vi "7-19-19 Decreasing temp.vi"() -> ()   [LabVIEW 2016]
uses:
  <userlib>/Levylab/LV to ITX/LVtoITX.lvclass
  <vilib>/Analysis/NI_AALPro.lvlib
panel:
  out "G Vs Time 2":cluster{"Data":dbl[], "Data":dbl[]}(graph)
  in  "Path 2":path=path "G:/My Drive/Data/300 275 dec/SA40060.20190715.000007.dat"
  out "Data 2":dbl[][](array[numeric])
  out "dG/dt Vs Temp Normalized vs prev":cluster{"Data":dbl[], "Data":dbl[]}[](graph)
  out "dG/dt Vs Temp Normalized vs 275K":cluster{"Data":dbl[], "Data":dbl[]}[](graph)
  out "G Vs Time Fit":cluster{"Data":dbl[], "Data":dbl[]}[](graph)
  out "G Vs Time Cut":cluster{"Data":dbl[], "Data":dbl[]}[](graph)
  out "G Vs Temp":cluster{"Data":dbl[], "Data":dbl[]}[](graph)
  out "Data":dbl[][](array[numeric])
  out "G Vs Time":cluster{"Data":dbl[], "Data":dbl[]}[](graph)
  out "Wavenames":string[](array[string])
  in  "Path":path=path "G:/My Drive/Data/300 275 dec/SA40060.20190715.000007.dat"
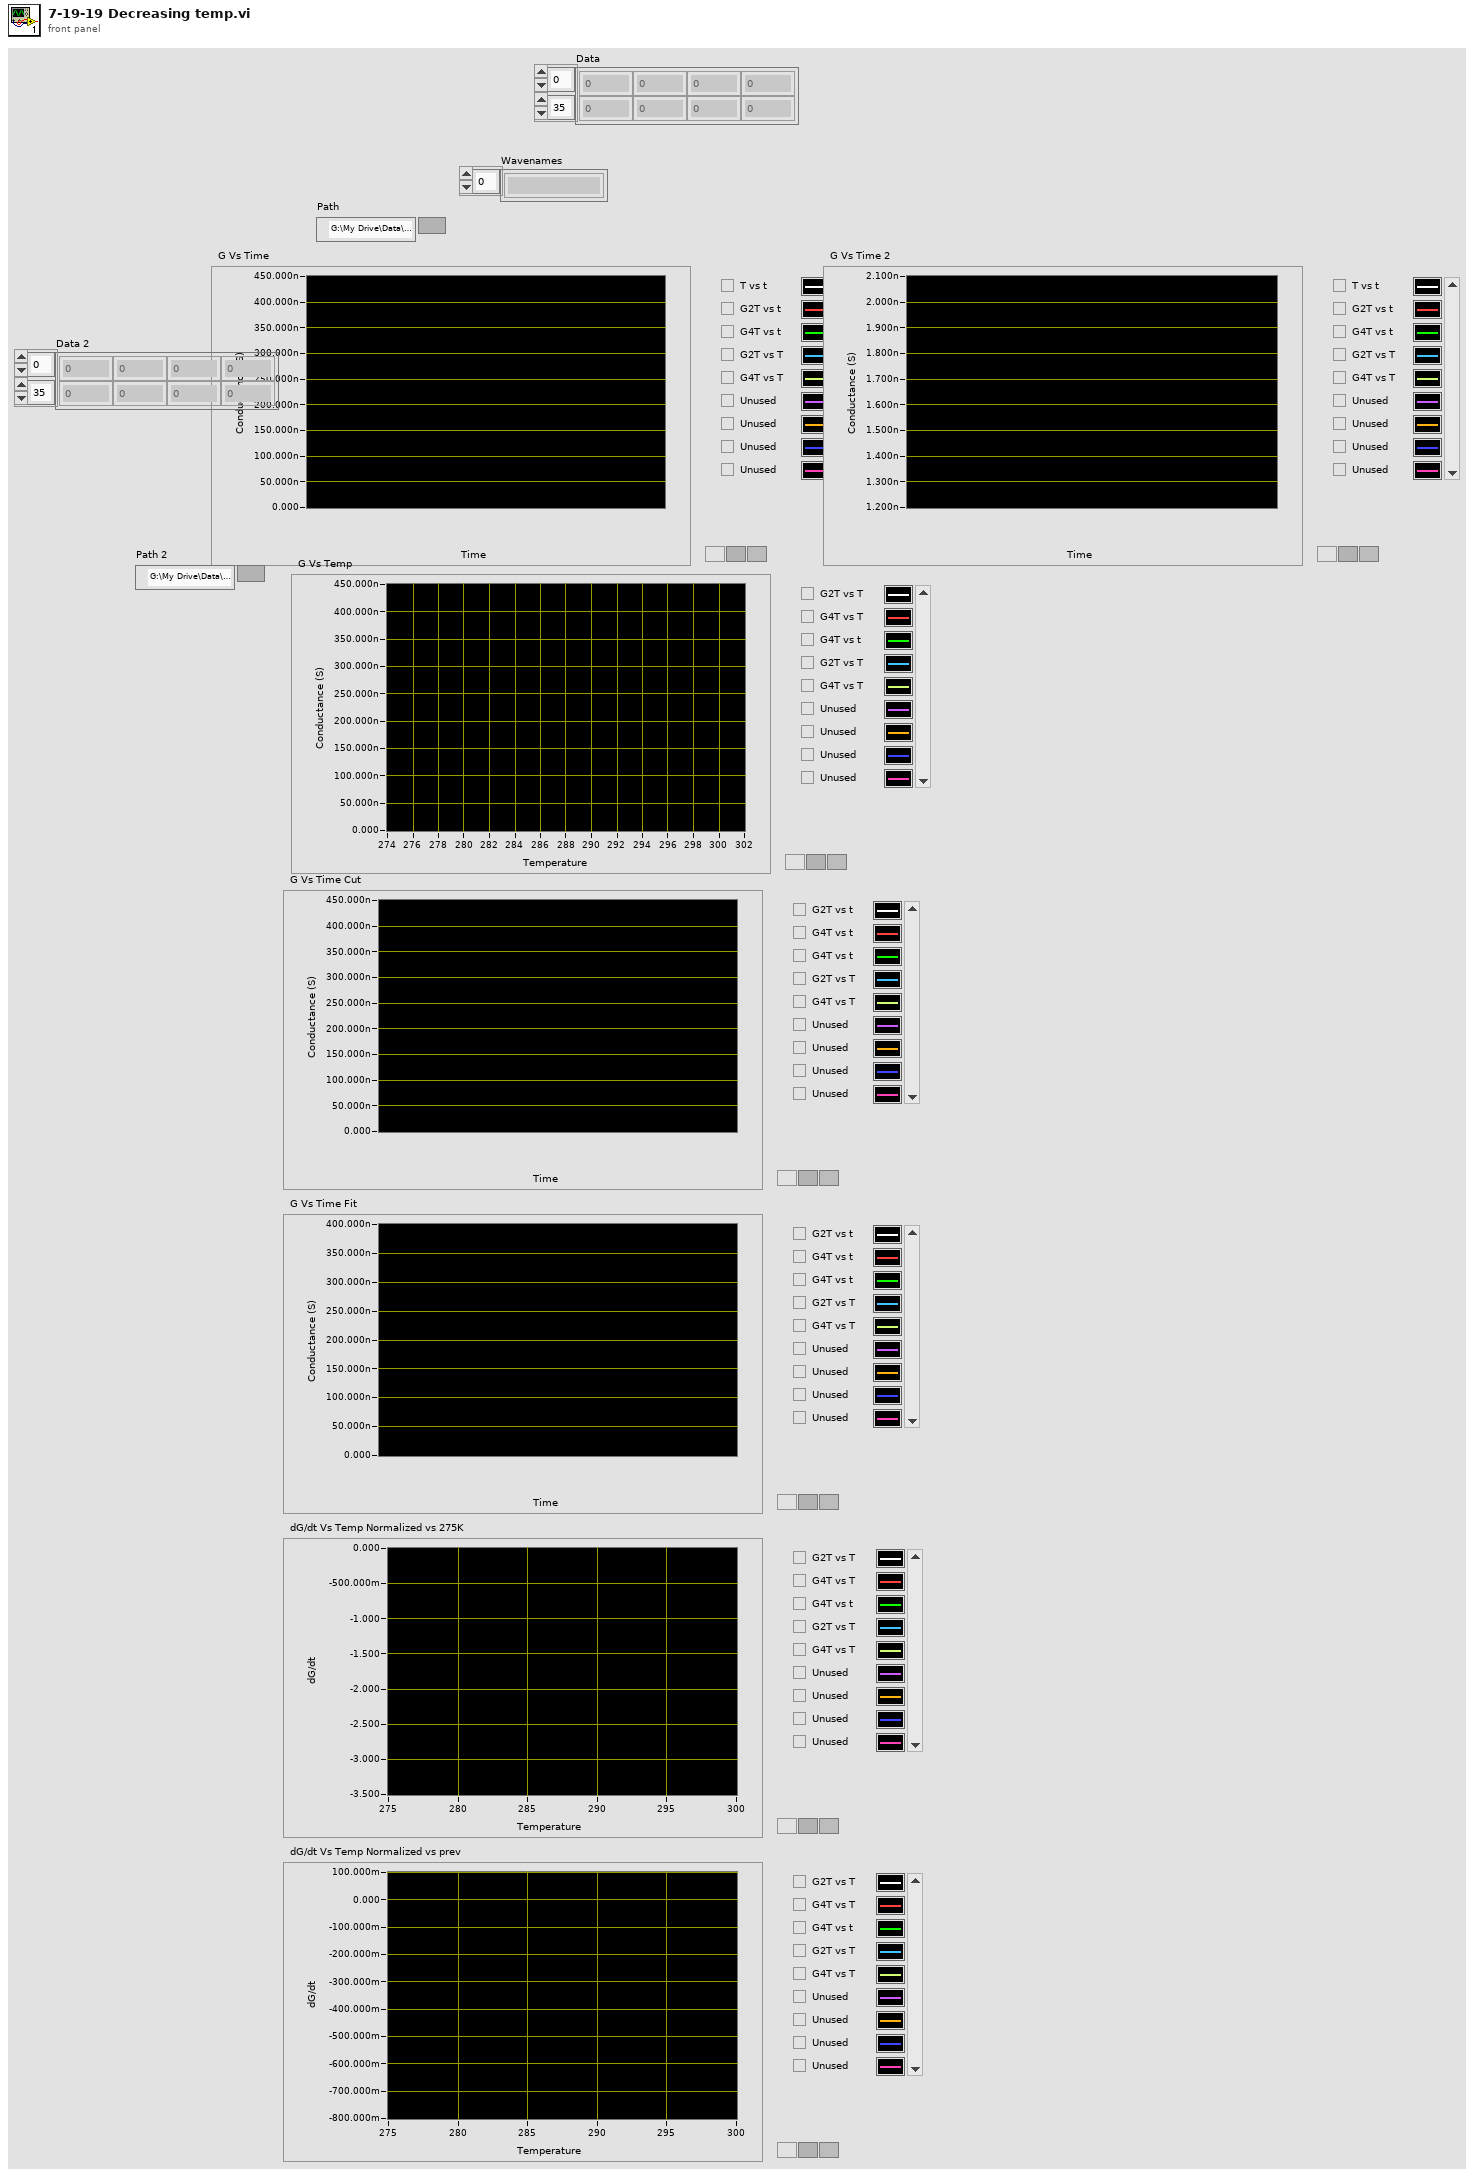
[diagram p1: front panel]
types:
  T1 = cluster{"slope min":dbl, "slope max":dbl, "intercept min":dbl, "intercept max":dbl}
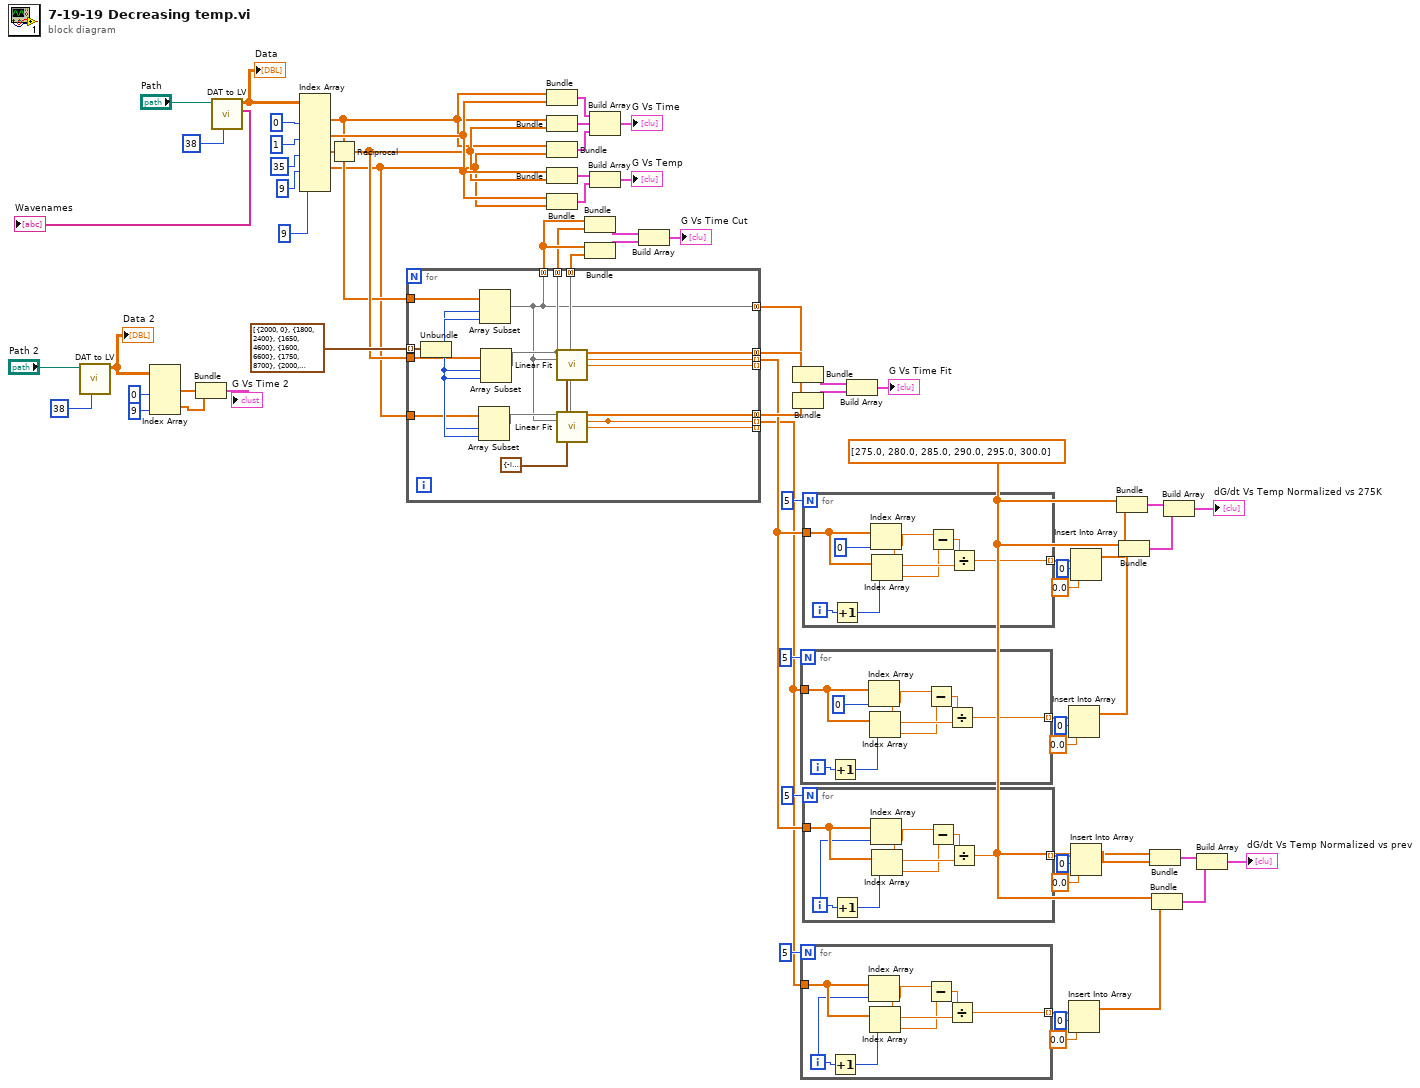
[diagram p0: block diagram]
diagram:
  w12 = dbl[] [275.0, 280.0, 285.0, 290.0, 295.0, 300.0]
  n1 = call <userlib>:"DAT to LV.vi"("header length"=38, "File Path"="Path 2") -> ("Data"=w6:dbl[][])  [unwired: 6 in, 3 out]
  "Data 2" <- w6
  n2 = Index Array(array=w6, index (col) #1=0 ("disabled index (col)"), index (col) #2=9 ("index (col)")) -> (element #1=w5:dbl[], element #2=w1:dbl[])  [unwired: 2 in]
  n3 = Bundle("Data"=w5, "Data"=w1) -> (→"G Vs Time 2":cluster{"Data":dbl[], "Data":dbl[]})  [unwired: 1 in]
  n4 = call <userlib>:"DAT to LV.vi"("header length"=38, "File Path"="Path") -> ("Wavenames"=→"Wavenames":string[], "Data"=w68:dbl[][])  [unwired: 6 in, 2 out]
  "Data" <- w68
  n5 = Index Array(array=w68, index (col) #1=0 ("disabled index (col)"), index (col) #2=1 ("index (col)"), index (col) #3=35 ("index (col)"), index (col) #4=9 ("index (col)"), index (col) #5=9 ("index (col)")) -> (element #1=w10:dbl[], element #2=w55:dbl[], element #3=w54:dbl[], element #4=w9:dbl[])  [unwired: 5 in, 1 out]
  n6 = Reciprocal(x=w54) -> (1/x=w47:dbl[])
  n7 = for {
    tunnel: cluster{"length":i32, "index":i32}[] [{"length"=2000, "index"=0}, {"length"=1800, "index"=2400}, {"length"=1650, "index"=4600}, {"length"=1600, "index"=6600}, {"length"=1750, "index"=8700}, {"length"=2000, "index"=10800}] -> [w87] mode=indexing
    tunnel: w10 -> [w84]
    tunnel: w47 -> [w83]
    tunnel: w9 -> [w82]
    tunnel: [w80] -> w43 mode=concatenating
    tunnel: [w79] -> w42 mode=concatenating
    tunnel: [w72] -> _ mode=indexing
    tunnel: [w78] -> _ mode=indexing
    tunnel: [w77] -> w15 mode=indexing
    tunnel: [w76] -> _ mode=indexing
    tunnel: [w73] -> w51 mode=concatenating
    tunnel: [w75] -> w50 mode=concatenating
    tunnel: [w74] -> w49 mode=concatenating
    tunnel: [w73] -> w13 mode=concatenating
    tunnel: [w72] -> w14 mode=indexing
    w81 = T1 {"slope min"=-inf, "slope max"=inf, "intercept min"=-inf, "intercept max"=inf} ("parameter bounds")
    n8 = Unbundle(w87) -> ("length"=w86:i32, "index"=w85:i32)
    n9 = Array Subset(array=w82, index=w85, length=w86) -> (w74:dbl[])
    n10 = Array Subset(array=w84, index=w85, length=w86) -> (w73:dbl[])
    n11 = Array Subset(array=w83, index=w85, length=w86) -> (w75:dbl[])
    n12 = call <vilib>:"Linear Fit.vi"("Y"=w75, "X"=w73, "parameter bounds"=w81) -> ("Best Linear Fit"=w80:dbl[], "slope"=w77:dbl, "intercept"=w76:dbl)  [unwired: 8 in, 2 out]
    n13 = call <vilib>:"Linear Fit.vi"("Y"=w74, "X"=w73, "parameter bounds"=w81) -> ("Best Linear Fit"=w79:dbl[], "slope"=w72:dbl, "intercept"=w78:dbl)  [unwired: 8 in, 2 out]
  }
  n14 = Bundle("Data"=w10, "Data"=w55) -> (w63:cluster{"Data":dbl[], "Data":dbl[]})  [unwired: 1 in]
  n15 = Bundle("Data"=w10, w47) -> (w62:cluster{"Data":dbl[], dbl[]})  [unwired: 1 in]
  n16 = Bundle("Data"=w10, "Data"=w9) -> (w61:cluster{"Data":dbl[], "Data":dbl[]})  [unwired: 1 in]
  n17 = Bundle("Data"=w55, w47) -> (w60:cluster{"Data":dbl[], dbl[]})  [unwired: 1 in]
  n18 = Bundle("Data"=w55, "Data"=w9) -> (w59:cluster{"Data":dbl[], "Data":dbl[]})  [unwired: 1 in]
  n19 = Bundle(w51, w50) -> (w52:cluster{dbl[], dbl[]})  [unwired: 1 in]
  n20 = Bundle(w51, w49) -> (w48:cluster{dbl[], dbl[]})  [unwired: 1 in]
  n21 = Build Array(w63, w62, w61) -> (→"G Vs Time":cluster{"Data":dbl[], "Data":dbl[]}[])
  n22 = Build Array(w60, w59) -> (→"G Vs Temp":cluster{"Data":dbl[], "Data":dbl[]}[])
  n23 = Build Array(w52, w48) -> (→"G Vs Time Cut":cluster{dbl[], dbl[]}[])
  n24 = Bundle(w13, "Best Linear Fit"=w43) -> (w45:cluster{dbl[], "Best Linear Fit":dbl[]})  [unwired: 1 in]
  n25 = Bundle(w13, "Best Linear Fit"=w42) -> (w46:cluster{dbl[], "Best Linear Fit":dbl[]})  [unwired: 1 in]
  n26 = for {
    N: 5 -> [_]
    tunnel: w14 -> [w95]
    tunnel: [w88] -> w33 mode=indexing
    i -> [w93]
    n27 = Increment(x=w93) -> (x+1=w92:i32)
    n28 = Index Array(array=w95, index=0) -> (element=w90:dbl)
    n29 = Index Array(array=w95, index=w92) -> (element=w89:dbl)
    n30 = Subtract(x=w90, y=w89) -> (x-y=w91:dbl)
    n31 = Divide(x=w91, y=w90) -> (x/y=w88:dbl)
  }
  n32 = for {
    N: 5 -> [_]
    tunnel: w14 -> [w102]
    tunnel: [w97] -> w27 mode=indexing
    i -> [w96]
    n33 = Increment(x=w96) -> (x+1=w101:i32)
    n34 = Index Array(array=w102, index=w96) -> (element=w99:dbl)
    n35 = Index Array(array=w102, index=w101) -> (element=w98:dbl)
    n36 = Subtract(x=w99, y=w98) -> (x-y=w100:dbl)
    n37 = Divide(x=w100, y=w99) -> (x/y=w97:dbl)
  }
  n38 = for {
    N: 5 -> [_]
    tunnel: w15 -> [w110]
    tunnel: [w103] -> w40 mode=indexing
    i -> [w108]
    n39 = Increment(x=w108) -> (x+1=w107:i32)
    n40 = Index Array(array=w110, index=0) -> (element=w105:dbl)
    n41 = Index Array(array=w110, index=w107) -> (element=w104:dbl)
    n42 = Subtract(x=w105, y=w104) -> (x-y=w106:dbl)
    n43 = Divide(x=w106, y=w105) -> (x/y=w103:dbl)
  }
  n44 = for {
    N: 5 -> [_]
    tunnel: w15 -> [w117]
    tunnel: [w112] -> w22 mode=indexing
    i -> [w111]
    n45 = Increment(x=w111) -> (x+1=w116:i32)
    n46 = Index Array(array=w117, index=w111) -> (element=w114:dbl)
    n47 = Index Array(array=w117, index=w116) -> (element=w113:dbl)
    n48 = Subtract(x=w114, y=w113) -> (x-y=w115:dbl)
    n49 = Divide(x=w115, y=w114) -> (x/y=w112:dbl)
  }
  n50 = Build Array(w45, w46) -> (→"G Vs Time Fit":cluster{dbl[], "Best Linear Fit":dbl[]}[])
  n51 = Insert Into Array(array=w33, index=0, new element=0.0 ("new element/subarray")) -> (w31:dbl[])
  n52 = Insert Into Array(array=w27, index=0, new element=0.0 ("new element/subarray")) -> (w17:dbl[])
  n53 = Insert Into Array(array=w40, index=0, new element=0.0 ("new element/subarray")) -> (w30:dbl[])
  n54 = Insert Into Array(array=w22, index=0, new element=0.0 ("new element/subarray")) -> (w16:dbl[])
  n55 = Bundle(w12, w30) -> (w37:cluster{dbl[], dbl[]})  [unwired: 1 in]
  n56 = Bundle(w12, w31) -> (w36:cluster{dbl[], dbl[]})  [unwired: 1 in]
  n57 = Bundle(w12, w16) -> (w18:cluster{dbl[], dbl[]})  [unwired: 1 in]
  n58 = Bundle(w12, w17) -> (w19:cluster{dbl[], dbl[]})  [unwired: 1 in]
  n59 = Build Array(w37, w36) -> (→"dG/dt Vs Temp Normalized vs 275K":cluster{dbl[], dbl[]}[])
  n60 = Build Array(w18, w19) -> (→"dG/dt Vs Temp Normalized vs prev":cluster{dbl[], dbl[]}[])
